vi "Parse URI.vi"(10 "error in (no error)":errorcluster, 11 "URI String":string) -> (2 "error out":errorcluster, 3 "Parsed Components":T1)   [LabVIEW 2020, in "URI.lvlib"]
uses:
  URI.lvlib
  URI Components.ctl
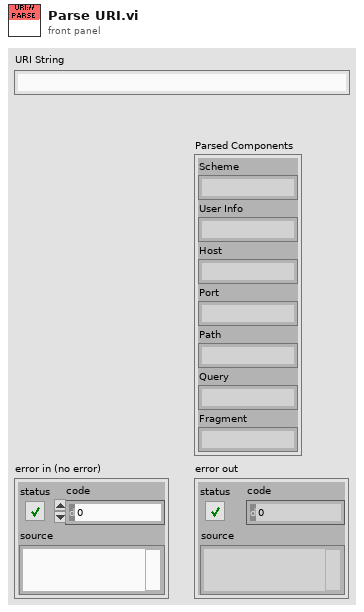
[diagram p1: front panel]
types:
  T1 = typedef "URI.lvlib/URI Components.ctl" = cluster{"Scheme":string, "User Info":string, "Host":string, "Port":string, "Path":string, "Query":string, "Fragment":string}
  T2 = typedef "URI.lvlib/Authority.ctl" = cluster{"Host":string, "Port":string, "User Info":string}
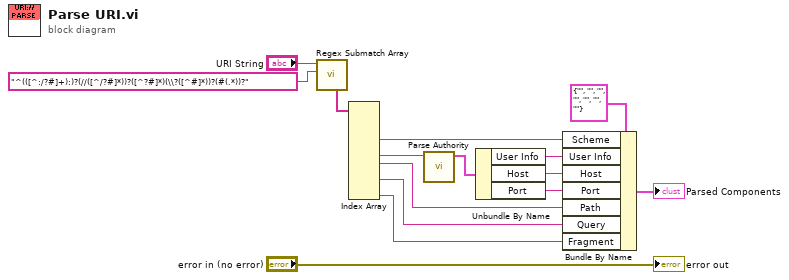
[diagram p0: block diagram]
diagram:
  n1 = call "Regex Submatch Array.vi"("regular expression"="^(([^:/?#]+):)?(//([^/?#]*))?([^?#]*)(\\?([^#]*))?(#(.*))?", "string"="URI String") -> ("matches"=w5:string[])  [unwired: 5 in, 4 out]
  n2 = Index Array(array=w5) -> (element #3=w8:string, element #5=w4:string, element #6=w3:string, element #8=w2:string, element #10=w1:string)  [unwired: 10 in, 5 out]
  n3 = call "Parse Authority.vi"("Authority String"=w4) -> ("Authority"=w12:T2)  [unwired: 9 in, 1 out]
  n4 = Unbundle By Name(w12) -> ("User Info"=w11:string, "Host"=w10:string, "Port"=w9:string)
  n5 = Bundle By Name(cluster=T1 {"Scheme"="", "User Info"="", "Host"="", "Port"="", "Path"="", "Query"="", "Fragment"=""} ("URI Components"), "Scheme"=w8, "User Info"=w11, "Host"=w10, "Port"=w9, "Path"=w3, "Query"=w2, "Fragment"=w1) -> (→"Parsed Components":T1)
  "error out" <- "error in (no error)"
